vi "adsr_attack.vi"(6 "Attack":dbl(knob) scale=0.05..0.001, 8 "error in (no error)":errorcluster, 10 "Number of samples":i32, 11 "Current Amplitude":dbl) -> (0 "error out":errorcluster, 2 "Current amplitude":dbl, 3 "Ramp Pattern":dbl[](array[numeric]))   [LabVIEW 2024]
uses:
  <vilib>/Analysis/1siggen.llb/Ramp Pattern by Samples.vi
  <vilib>/Analysis/NI_AALBase.lvlib
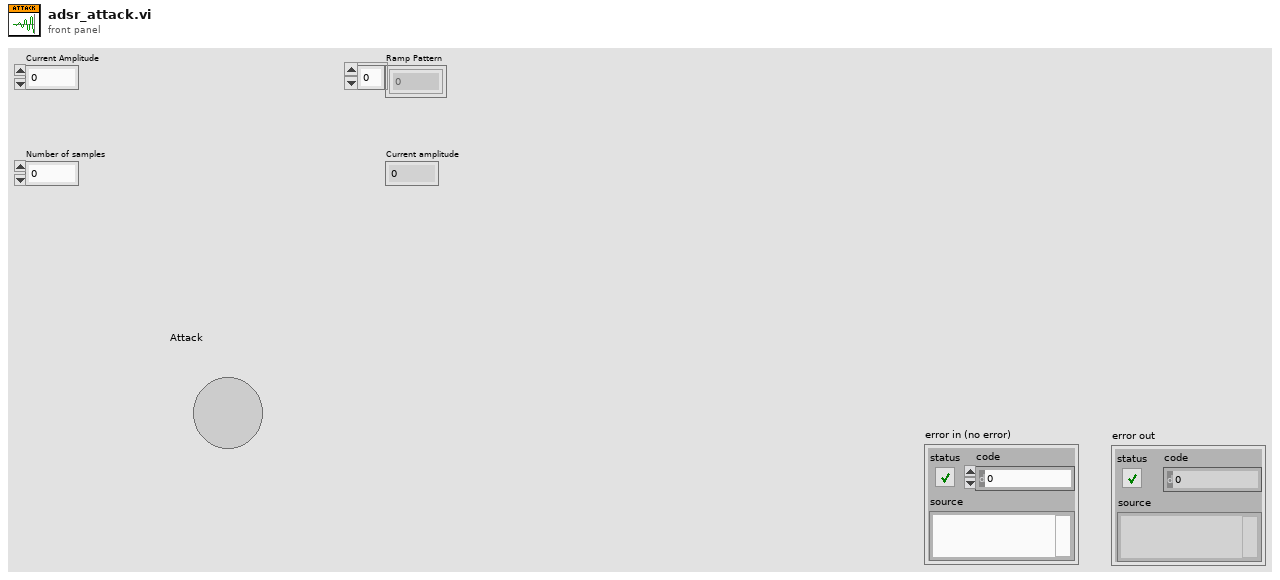
[diagram p1: front panel]
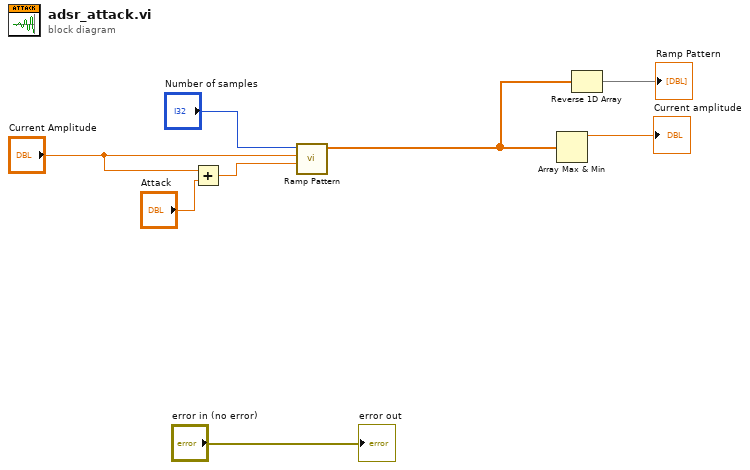
[diagram p0: block diagram]
diagram:
  n1 = Add(x="Current Amplitude", y="Attack") -> (x+y=w5:dbl)
  n2 = call-poly <vilib>:"Ramp Pattern.vi"("start"=w5, "end"="Current Amplitude", "samples"="Number of samples") -> ("Ramp Pattern"=w7:dbl[])  [unwired: 7 in, 1 out]
  n3 = Array Max & Min(array=w7) -> (max value=→"Current amplitude":dbl)  [unwired: 3 out]
  n4 = Reverse 1D Array(array=w7) -> (reversed array=→"Ramp Pattern":dbl[])
  "error out" <- "error in (no error)"
